vi "serial write macro.vi"(3 "String":string, 4 "Delay (ms)":i32=250, 5 "VISA resource name":refnum<visa-resource-name>) -> (0 "read buffer":string, 1 "error out":errorcluster, 2 "VISA resource name out":refnum<visa-resource-name>)   [LabVIEW 2014]
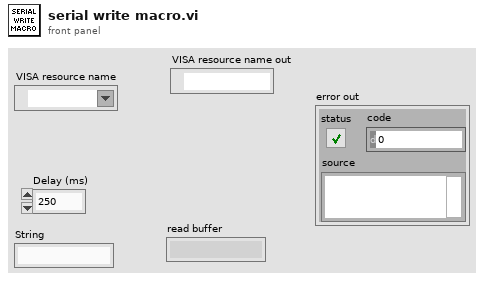
[diagram p1: front panel]
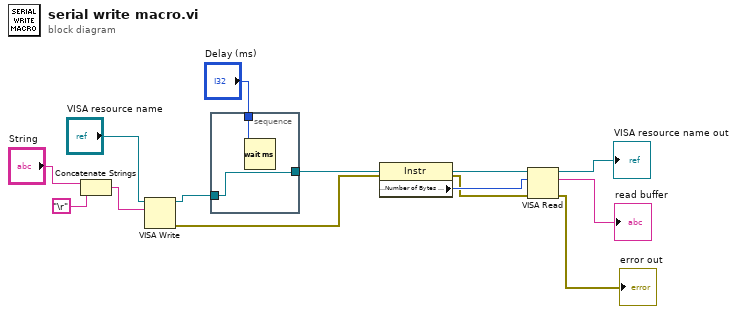
[diagram p0: block diagram]
diagram:
  n1 = Concatenate Strings("String", "\r") -> (w9:string)
  n2 = VISA Write(VISA resource name="VISA resource name", write buffer=w9) -> (VISA resource name out=w8:refnum<visa-resource-name>, error out=w7:errorcluster)  [unwired: 1 in, 1 out]
  n3 = stacked-sequence {
    tunnel: [w16] -> w14
    tunnel: w8 -> [w16]
    tunnel: "Delay (ms)" -> [w15]
    frame #0 {
      n4 = Wait (ms)(milliseconds to wait=w15) -> ()  [unwired: 1 out]
    }
  }
  n5 = property class="Instr"(reference=w14, error in=w7) -> (reference out=w13:refnum<visa-resource-name>, error out=w11:errorcluster, "Serial Settings:Number of Bytes at Serial Port"=w12:u32)
  n6 = VISA Read(VISA resource name=w13, byte count=w12, error in (no error)=w11) -> (VISA resource name out=→"VISA resource name out":refnum<visa-resource-name>, read buffer=→"read buffer":string, error out=→"error out":errorcluster)  [unwired: 1 out]
